vi "Format Client Request (Notification).vi"(8 "error in (no error)":errorcluster, 9 "id":string, 10 "JSON Value in":refnum<class "JSON Value.lvclass">, 11 "method":string) -> (0 "error out":errorcluster, 2 "Request String":string)   [LabVIEW 2016, in "JSONRPC Client.lvclass"]
uses:
  JSONRPC Client.lvclass
  <vilib>/NI/JSON Support for LabVIEW/JSON Value/JSON Value.lvclass
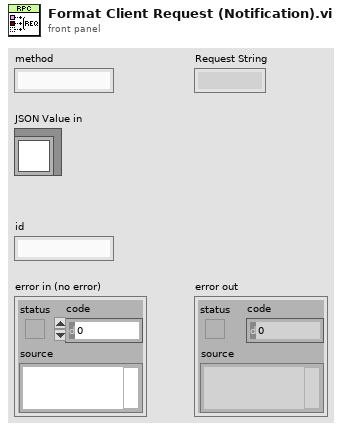
[diagram p1: front panel]
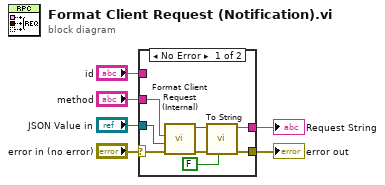
[diagram p0: block diagram]
diagram:
  n1 = case shown="No Error" "error in (no error)" {
    selector: "error in (no error)" -> [w14 w15]
    tunnel: [w13 w15] -> w5
    tunnel: "JSON Value in" -> [w8 _]
    tunnel: [w12 _] -> w3
    tunnel: "method" -> [w11 _]
    tunnel: "id" -> [_ _]
    frame No Error {
      n2 = call "Format Client Request (Internal).vi"("error in (no error)"=w14, "params"=w8, "method"=w11) -> ("error out"=w10:errorcluster, "JSON Value out"=w9:refnum<class "JSON Value.lvclass">)  [unwired: 7 in]
      n3 = call <vilib>:"To String.vi"("pretty print? (T)"=FALSE, "error in (no error)"=w10, "JSON Value in"=w9) -> ("error out"=w13:errorcluster, "String"=w12:string)  [unwired: 7 in]
    }
    frame Error {
    }
  }
  "error out" <- w5
  "Request String" <- w3
